vi "Add PV Monitors to FGV.vi"(8 "Error In":errorcluster, 10 "PV Monitor Section":string="PV_Monitors", 11 "CS++Factory":refnum<class "CS++Factory.lvclass">) -> (0 "Error Out":errorcluster)   [LabVIEW 2015, in "CS++ProcessVariables.lvlib"]
doc: "Read PV Monitors from configuration data to FGV."
uses:
  CS++ProcessVariables.lvlib
  CS++BaseClasses/Factory/CS++Factory.lvclass
  Libraries/Base/FGV Action.ctl
  Actors/CS++PVMonitor/CS++PVMonitor.lvclass
  Libraries/Base/CS++Base.lvlib
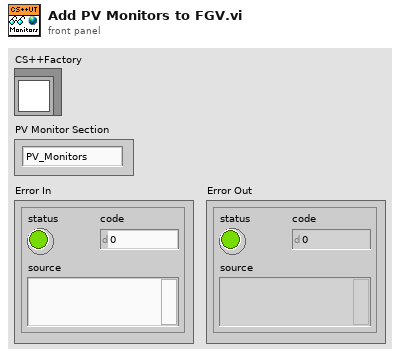
[diagram p1: front panel]
types:
  T1 = typedef "CS++Base.lvlib/FGV Action.ctl" = enum16{"add", "replace", "read", "remove", "reset", "get attributes"}
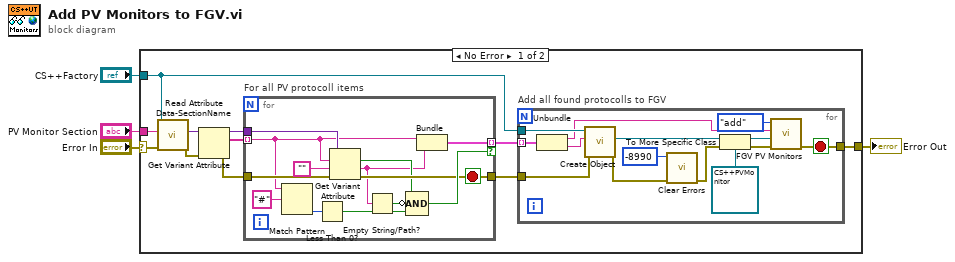
[diagram p0: block diagram]
diagram:
  n1 = case shown="No Error" "Error In" {
    selector: "Error In" -> [w5 w43]
    tunnel: "PV Monitor Section" -> [w8 _]
    tunnel: "CS++Factory" -> [w9 _]
    tunnel: [w10 w43] -> w2
    frame No Error {
      n2 = call-dynamic "Read Attribute Data-SectionName.vi"("error in (no error)"=w5, "Object Name"=w8, "CS++Factory in"=w9) -> ("error out"=w6:errorcluster, "Attribute Data"=w7:variant)  [unwired: 6 in, 1 out]
      n3 = Get Variant Attribute(Variant=w7, error in=w6) -> (duplicate Variant=w14:variant, names=w15:string[], error out=w13:errorcluster)  [unwired: 2 in, 1 out]
      n4 = for "For all PV protocoll items" {
        tunnel: w15 -> [w38] mode=indexing
        tunnel: [w40] -> w11 mode=indexing if=w39
        tunnel: w14 -> [w42]
        tunnel: w13 -> [w41]
        tunnel: [w37] -> w12
        stop <- w37 stop-if-true
        n5 = Match Pattern(string=w38, regular expression="#") -> (offset past match=w35:i32)  [unwired: 1 in, 3 out]
        n6 = Less Than 0?(x=w35) -> (x < 0?=w34:bool)
        n7 = Get Variant Attribute(Variant=w42, name=w38, default value (empty Variant)="", error in=w41) -> (found=w32:bool, value=w30:string, error out=w37:errorcluster)  [unwired: 1 out]
        n8 = Empty String/Path?(string/path=w30) -> (empty?=w31:bool)
        n9 = Compound Arithmetic op=AND(w32, invert w31, w34) -> (w39:bool)
        n10 = Bundle(w38, w30) -> (w40:cluster{string, string})  [unwired: 1 in]
      }
      n11 = for "Add all found protocolls to FGV" {
        tunnel: w12 -> [w26]
        tunnel: w11 -> [w29] mode=indexing
        tunnel: w9 -> [w28]
        tunnel: [w21] -> w10
        stop <- w21 stop-if-true
        n12 = Unbundle(w29) -> (w20:string, w19:string)
        n13 = call "Create Object.vi"("error in (no error)"=w26, "Object Name"=w19, "CS++Factory in"=w28) -> ("error out"=w17:errorcluster, "LabVIEW Object"=w27:refnum<class>)  [unwired: 5 in, 2 out]
        n14 = call <vilib>:"Clear Errors.vi"("error in (no error)"=w17, "specific error code to clear (0: all)"=-8990) -> ("error out"=w16:errorcluster)  [unwired: 4 in, 1 out]
        n15 = To More Specific Class(target class=refnum<class "CS++PVMonitor.lvclass"> refnum ("CS++PVMonitor.lvlib:CS++PVMonitor.lvclass"), reference=w27, error in=w16) -> (specific class reference=w23:refnum<class "CS++PVMonitor.lvclass">, error out=w22:errorcluster)
        n16 = call "FGV PV Monitors.vi"("Error In"=w22, "CS++PVMonitor"=w23, "PV Monitor"=w20, "Action (read)"=FGV_Action."add") -> ("Error Out"=w21:errorcluster)  [unwired: 3 in, 4 out]
      }
    }
    frame Error {
    }
  }
  "Error Out" <- w2
